vi "ConfocalMode.vi"() -> ()   [LabVIEW 2010]
panel:
  in  "Confocal Mode Area Image calculation":enum32{"Maximum", "Average", "Normalized"}(ring)
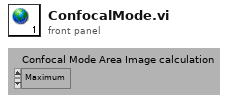
[diagram p1: front panel]
diagram:
